vi "MCLB Update Cell.vi"(8 "error in (no error)":errorcluster, 11 "View in":refnum<class "MCListbox View.lvclass">) -> (0 "error out":errorcluster, 1 "Active Cell":T1, 2 "Value":string, 3 "View out":refnum<class "MCListbox View.lvclass">, 5 "Update?":bool)   [LabVIEW 2013, in "SET Project Editor.lvlib" / "MCListbox View.lvclass"]
uses:
  MCListbox View.lvclass
  <vilib>/Utility/miscctls.llb/LVRowAndColumnTypeDef.ctl
  MCListbox View.lvclass/MCListbox View.ctl
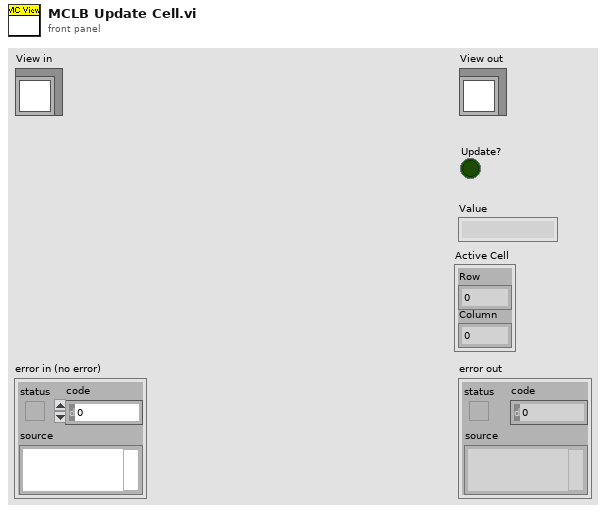
[diagram p1: front panel]
types:
  T1 = typedef "LVRowAndColumnTypeDef.ctl" = cluster{"Row":i32, "Column":i32}
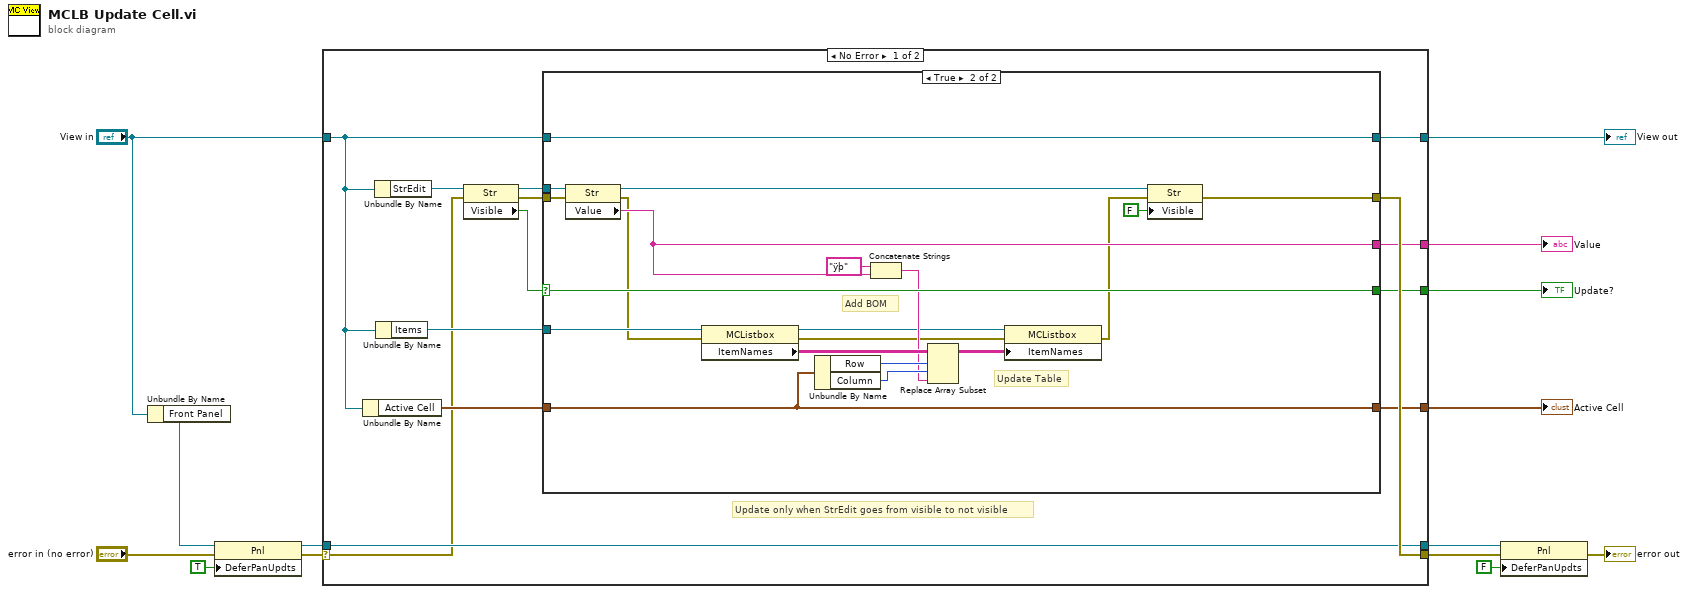
[diagram p0: block diagram]
diagram:
  n1 = Unbundle By Name("View in") -> ("Front Panel"=w12:refnum<vi>)
  n2 = property class="Pnl"(reference=w12, error in="error in (no error)", "DeferPanUpdts"=TRUE ("Defer Panel Updates")) -> (reference out=w8:refnum<vi>, error out=w9:errorcluster)
  n3 = case shown="No Error" w9 {
    selector: w9 -> [w17 w54]
    tunnel: [w21 w54] -> w6
    tunnel: [w23 w53] -> w14
    tunnel: "View in" -> [w22 w53]
    tunnel: w8 -> [w20 w52]
    tunnel: [w20 w52] -> w7
    tunnel: [w19 _] -> w2
    tunnel: [w18 _] -> w3
    tunnel: [w15 _] -> w1
    frame No Error {
      # "Update only when StrEdit goes from visible to not visible"
      n4 = Unbundle By Name(w22) -> ("Active Cell"=w24:T1)
      n5 = Unbundle By Name(w22) -> ("StrEdit"=w28:refnum<vi>)
      n6 = Unbundle By Name(w22) -> ("Items"=w25:refnum<vi>)
      n7 = property class="Str"(reference=w28, error in=w17) -> (reference out=w26:refnum<vi>, error out=w16:errorcluster, "Visible"=w27:bool)
      n8 = case shown="True" w27 {
        selector: w27 -> [_ w45]
        tunnel: w26 -> [_ w50]
        tunnel: w25 -> [_ w43]
        tunnel: w22 -> [w31 w47]
        tunnel: [w30 w48] -> w21
        tunnel: [w31 w47] -> w23
        tunnel: w24 -> [w29 w44]
        tunnel: [_ w39] -> w19
        tunnel: [w29 w44] -> w18
        tunnel: w16 -> [w30 w46]
        tunnel: [_ w45] -> w15
        frame False {
        }
        frame True {
          # "Update Table"
          # "Add BOM"
          n9 = property class="Str"(reference=w50, error in=w46) -> (reference out=w49:refnum<vi>, error out=w34:errorcluster, "Value"=w39:string)
          n10 = property class="MCListbox"(reference=w43, error in=w34) -> (reference out=w35:refnum<vi>, error out=w33:errorcluster, "ItemNames"=w42:string[][])
          n11 = Unbundle By Name(w44) -> ("Row"=w41:i32, "Column"=w40:i32)
          n12 = Concatenate Strings("ÿþ" ("string"), w39) -> (w37:string)
          n13 = Replace Array Subset(array=w42, new element=w37, index (row)=w41, index (col)=w40) -> (w36:string[][])
          n14 = property class="MCListbox"(reference=w35, error in=w33, "ItemNames"=w36) -> (error out=w32:errorcluster)  [unwired: 1 out]
          n15 = property class="Str"(reference=w49, error in=w32, "Visible"=FALSE) -> (error out=w48:errorcluster)  [unwired: 1 out]
        }
      }
    }
    frame Error {
    }
  }
  "View out" <- w14
  "Active Cell" <- w3
  "Value" <- w2
  "Update?" <- w1
  n16 = property class="Pnl"(reference=w7, error in=w6, "DeferPanUpdts"=FALSE ("Defer Panel Updates")) -> (error out=→"error out":errorcluster)  [unwired: 1 out]
